vi "Flood-Water level detector.vi"() -> ()   [LabVIEW 2021]
panel:
  out "Water Level > Max3 (High 170 cm)":bool
  out "Water Level > Max2 (High 150 cm)":bool
  out "Water Level > Max1 (High 140 cm)":bool
  out "cm":dbl
  out "cm":dbl(slide) scale=0.0..200.0
  out "Water Level Monitoring":dynamicdata(graph)
  in  "Data":dbl
  in  "stop":bool
  in  "Tab Control":enum32{"Page 1", "Page 2"}(tab)
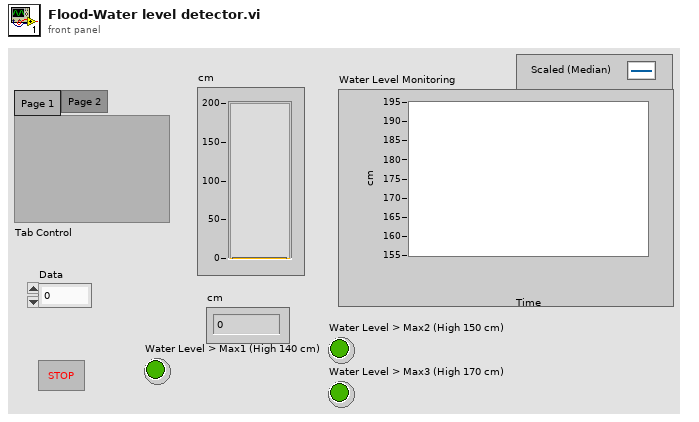
[diagram p1: front panel]
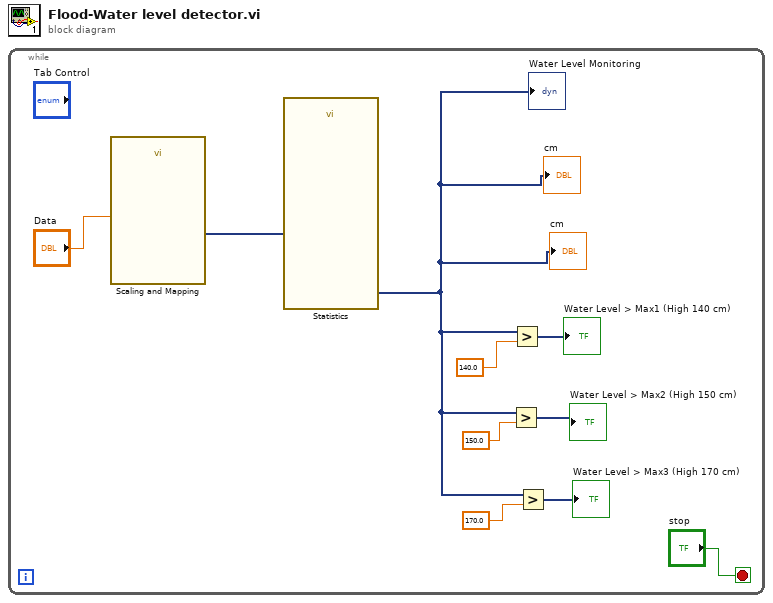
[diagram p0: block diagram]
diagram:
  n1 = while {
    stop <- "stop" stop-if-true
    n2 = call "Scaling and Mapping"("Signals"="Data") -> ("Scaled Signals"=w9:dynamicdata)  [unwired: 9 in, 1 out]
    n3 = call "Statistics"("Signals"=w9) -> ("Median"=w4:dynamicdata)  [unwired: 16 in, 10 out]
    "Water Level Monitoring" <- w4
    "cm" <- w4
    "cm" <- w4
    n4 = Greater?(x=w4, y=150.0) -> (0:→"Water Level > Max2 (High 150 cm)":dynamicdata)
    n5 = Greater?(x=w4, y=140.0) -> (0:→"Water Level > Max1 (High 140 cm)":dynamicdata)
    n6 = Greater?(x=w4, y=170.0) -> (0:→"Water Level > Max3 (High 170 cm)":dynamicdata)
  }
